vi "Pre Launch Init.vi"(11 "Car Wash Controller in":refnum<class "Vehicle Position Simulation Actor.lvclass">) -> (0 "error out":errorcluster, 3 "Car Wash Controller out":refnum<class "Vehicle Position Simulation Actor.lvclass">)   [LabVIEW 2019, in "Vehicle Position Sinmulation Actor.lvlib" / "Vehicle Position Simulation Actor.lvclass"]
doc: "(<B>Filename</B>: Actor Framework.lvlib:Actor.lvclass:Pre Launch Init.vi)\n\nDefines behavior that occurs after the Launch Nested Actor method is invoked but before the actor's Actor Core method begins running.\n\nBy default, this method does nothing. A descendant class may override it to define behavior."
uses:
  Vehicle Position Simulation Actor.lvclass
  Vehicle Position Simulation Actor.lvclass/Vehicle Position Simulation Actor.ctl
  Vehicle Position Interface/Vehicle Position Interface/Vehicle Position Interface.lvclass
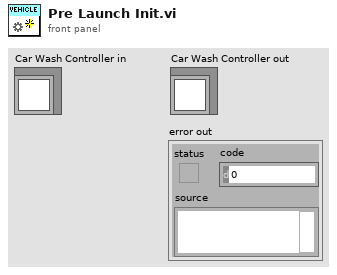
[diagram p1: front panel]
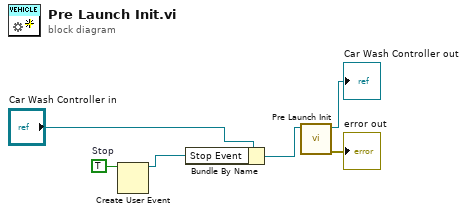
[diagram p0: block diagram]
diagram:
  w4 = TRUE  # Stop
  n1 = Create User Event(user event datatype=w4) -> (user event=w2:refnum<user-event>)  [unwired: 1 in, 1 out]
  n2 = Bundle By Name(cluster="Car Wash Controller in", "Stop Event"=w2) -> (w1:refnum<class "Vehicle Position Simulation Actor.lvclass">)
  n3 = call-parent "Pre Launch Init.vi"("Actor in"=w1) -> ("error out"=→"error out":errorcluster, "Actor out"=→"Car Wash Controller out":refnum<class "Vehicle Position Simulation Actor.lvclass">)  [unwired: 9 in]
